vi "LogRX.vi"(8 "error in (no error)":errorcluster, 11 "Stream in":refnum<class "Stream.lvclass">) -> (0 "error out":errorcluster, 3 "Stream out":refnum<class "Stream.lvclass">)   [LabVIEW 2018, in "Stream.lvclass"]
uses:
  Stream.lvclass
  Stream.lvclass/Stream.ctl
  Log/Log.lvclass
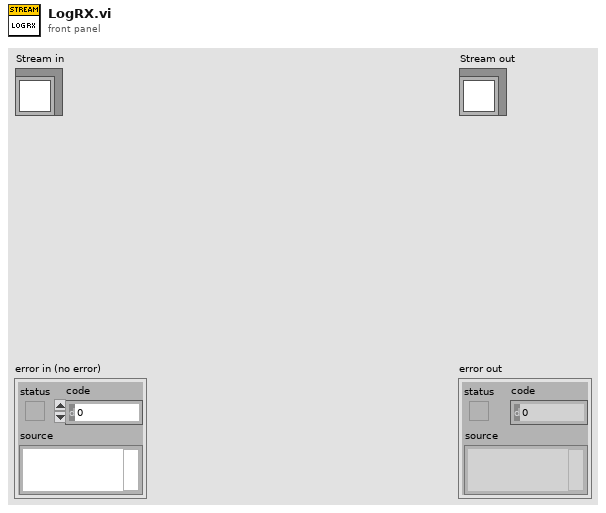
[diagram p1: front panel]
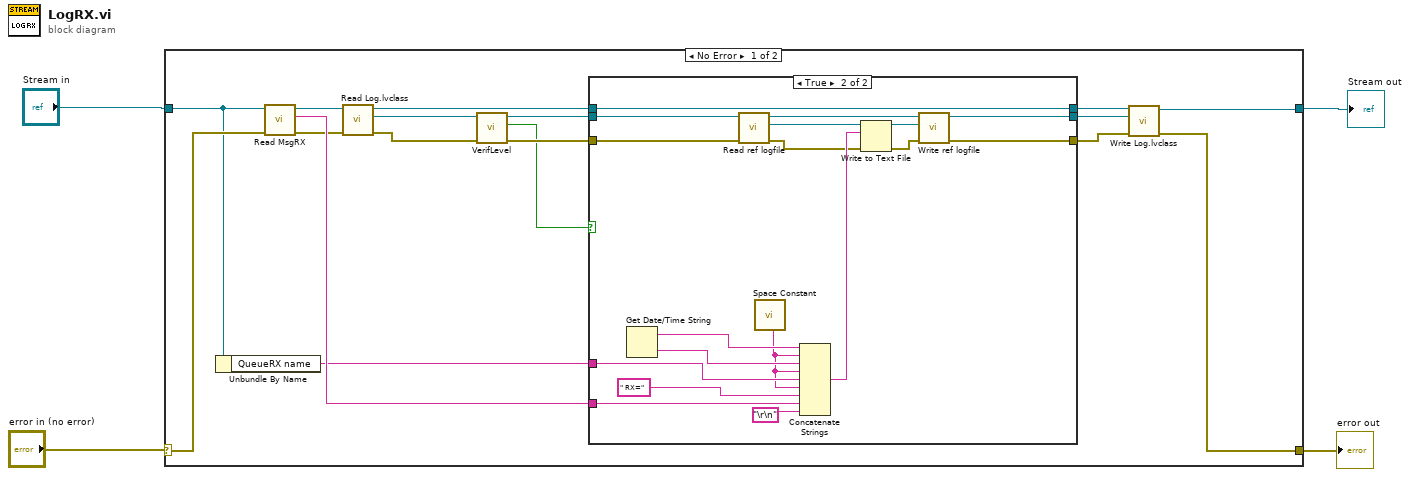
[diagram p0: block diagram]
diagram:
  n1 = case shown="No Error" "error in (no error)" {
    selector: "error in (no error)" -> [w21 w44]
    tunnel: [w5 w44] -> w2
    tunnel: [w6 w43] -> w3
    tunnel: "Stream in" -> [w19 w43]
    frame No Error {
      n2 = Unbundle By Name(w19) -> ("QueueRX name"=w18:string)
      n3 = call-dynamic "Read MsgRX.vi"("error in (no error)"=w21, "Comm in"=w19) -> ("error out"=w15:errorcluster, "MsgRX"=w20:string, "Comm out"=w17:refnum<class "Stream.lvclass">)  [unwired: 7 in]
      n4 = call-dynamic "Read Log.lvclass.vi"("error in (no error)"=w15, "Comm in"=w17) -> ("error out"=w12:errorcluster, "Log.lvclass"=w14:refnum<class "Log.lvclass">, "Comm out"=w16:refnum<class "Stream.lvclass">)  [unwired: 7 in]
      n5 = call-dynamic "VerifLevel.vi"("error in (no error)"=w12, "Log in"=w14) -> ("error out"=w11:errorcluster, "logging"=w10:bool, "Log out"=w13:refnum<class "Log.lvclass">)  [unwired: 7 in]
      n6 = case shown="True" w10 {
        tunnel: w16 -> [w24 w27]
        tunnel: w11 -> [w23 w29]
        tunnel: w20 -> [_ w39]
        tunnel: [w23 w26] -> w7
        tunnel: [w24 w27] -> w8
        tunnel: w18 -> [_ w36]
        tunnel: w13 -> [w22 w28]
        tunnel: [w22 w25] -> w9
        frame False {
        }
        frame True {
          n7 = Get Date/Time String() -> (date string=w42:string, time string=w41:string)  [unwired: 3 in]
          n8 = call-dynamic "Read ref logfile.vi"("error in (no error)"=w29, "Log in"=w28) -> ("error out"=w31:errorcluster, "ref logfile"=w34:refnum<file>, "Log out"=w32:refnum<class "Log.lvclass">)  [unwired: 7 in]
          n9 = call <vilib>:"Space Constant.vi"() -> ("String"=w35:string)
          n10 = Concatenate Strings(w42, w35, w41, w35, w36, w35, " RX=" ("string"), w39, "\r\n" ("string")) -> (w37:string)
          n11 = Write to Text File(file (use dialog)=w34, text=w37, error in=w31) -> (refnum out=w33:refnum<file>, error out=w30:errorcluster)  [unwired: 1 in, 1 out]
          n12 = call-dynamic "Write ref logfile.vi"("error in (no error)"=w30, "ref logfile"=w33, "Log in"=w32) -> ("error out"=w26:errorcluster, "Log out"=w25:refnum<class "Log.lvclass">)  [unwired: 7 in]
        }
      }
      n13 = call-dynamic "Write Log.lvclass.vi"("error in (no error)"=w7, "Log.lvclass"=w9, "Comm in"=w8) -> ("error out"=w5:errorcluster, "Comm out"=w6:refnum<class "Stream.lvclass">)  [unwired: 7 in]
    }
    frame Error {
    }
  }
  "error out" <- w2
  "Stream out" <- w3
